vi "Read Actor Core VI Ref.vi"(11 "AMS Gas Actor in":refnum<class "AMS Gas Actor.lvclass">) -> (2 "Actor Core VI Ref":refnum<vi>, 3 "AMS Gas Actor out":refnum<class "AMS Gas Actor.lvclass">)   [LabVIEW 2015, in "AMS UI.lvlib" / "AMS Gas Actor.lvclass"]
uses:
  AMS Gas Actor.lvclass
  AMS Gas Actor.lvclass/AMS Gas Actor.ctl
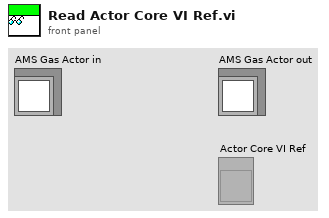
[diagram p1: front panel]
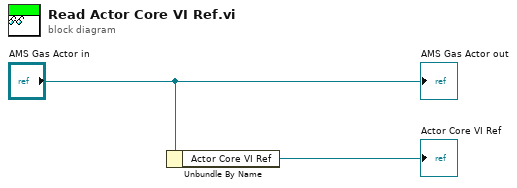
[diagram p0: block diagram]
diagram:
  n1 = Unbundle By Name("AMS Gas Actor in") -> ("Actor Core VI Ref"=→"Actor Core VI Ref":refnum<vi>)
  "AMS Gas Actor out" <- "AMS Gas Actor in"
